vi "FTW-Actor-HandleError.vi"(0 "FTW Actor Instance":refnum<class "FTW-ActorExtended.lvclass">, 5 "Explanation":string, 11 "error in":errorcluster) -> (4 "FTW Actor Instance out":refnum<class "FTW-ActorExtended.lvclass">, 6 "Exception occured?":T1, 8 "Serialized Event":string, 15 "error out":errorcluster)   [LabVIEW 2015, in "FTW-ActorExtended.lvclass"]
uses:
  FTW-ActorExtended.lvclass
  Error/FTW-ERR-ExceptionType.ctl
  FTW-ActorExtended.lvclass/FTW-ActorExtended.ctl
  Instance/FTW-ActorInstance.lvclass
panel:
  # "Inputs"
  # "Outputs"
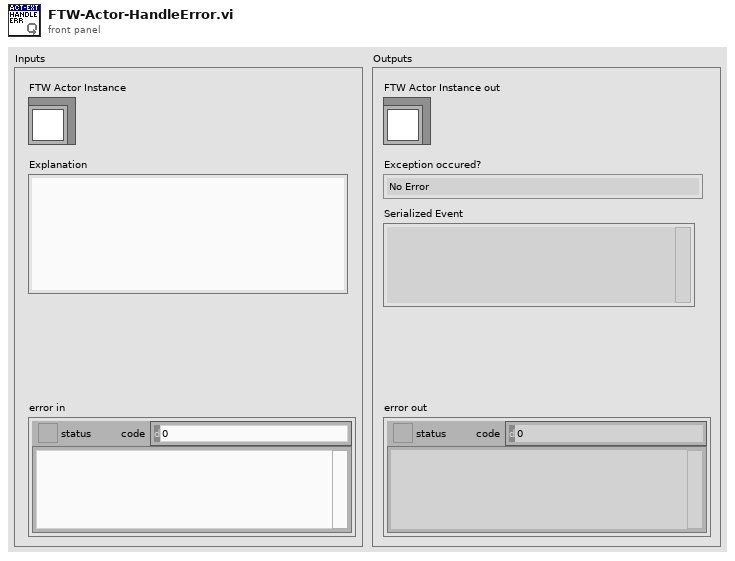
[diagram p1: front panel]
types:
  T1 = typedef "FTW-ERR-ExceptionType.ctl" = enum16{"No Error", "Error", "Warning"}
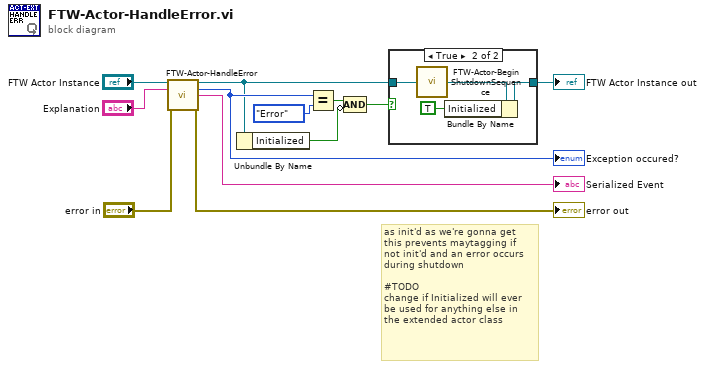
[diagram p0: block diagram]
diagram:
  # "as init'd as we're gonna get\nthis prevents maytagging if\nnot init'd and an error occurs\nduring shutdown\n\n#TODO\nchange if Initialized will ever\nbe used for anything else in\nthe extended actor class"
  n1 = call-parent "FTW-Actor-HandleError.vi"("FTW Actor Instance"="FTW Actor Instance", "Explanation"="Explanation", "error in"="error in") -> ("FTW Actor Instance out"=w5:refnum<class "FTW-ActorExtended.lvclass">, "Exception occured?"=w7:T1, "Serialized Event"=→"Serialized Event":string, "error out"=→"error out":errorcluster)  [unwired: 9 in]
  "Exception occured?" <- w7
  n2 = Unbundle By Name(w5) -> ("Initialized"=w4:bool)
  n3 = Equal?(x=w7, y=FTW-ERR-ExceptionType."Error") -> (x = y?=w3:bool)
  n4 = Compound Arithmetic op=AND(w3, invert w4) -> (w1:bool)
  n5 = case shown="True" w1 {
    tunnel: w5 -> [w13 w17]
    tunnel: [w13 w15] -> w2
    frame False {
    }
    frame True {
      n6 = call "FTW-Actor-BeginShutdownSequence.vi"("FTW Actor Instance"=w17) -> ("FTW Actor Instance out"=w16:refnum<class "FTW-ActorExtended.lvclass">)  [unwired: 3 in]
      n7 = Bundle By Name(cluster=w16, "Initialized"=TRUE) -> (w15:refnum<class "FTW-ActorExtended.lvclass">)
    }
  }
  "FTW Actor Instance out" <- w2
